vi "stupid get action.vi"(7 "transmit queue":refnum<queue>, 11 "application request in":T1) -> (0 "connection error":errorcluster)   [LabVIEW 2013]
uses:
  HTTP server/http request.ctl
  HTTP server/http method.ctl
  HTTP headers/http header data.ctl
  HTTP server/http response.ctl
  HTTP server/http response packet type.ctl
  HTTP server/Basic HTTP server.lvclass
  HTTP headers/http headers.lvlib
  HTTP responder/http responder.lvclass
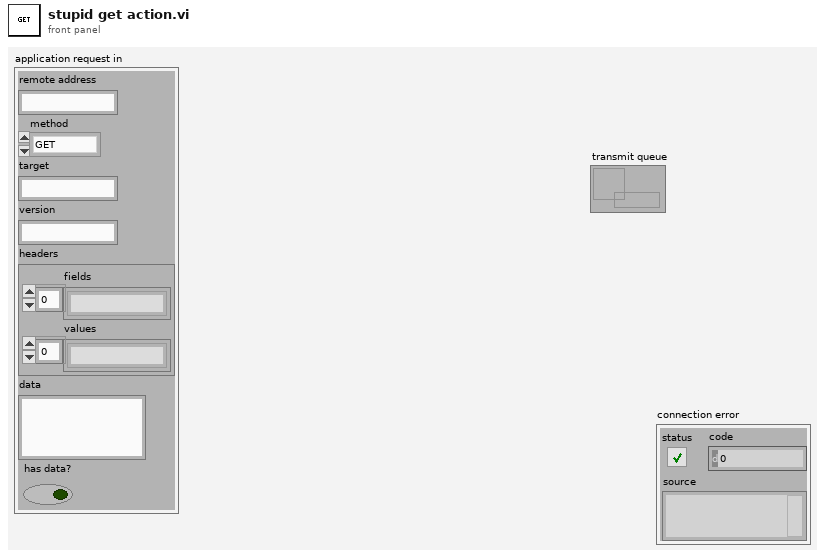
[diagram p1: front panel]
types:
  T1 = typedef "Basic HTTP server.lvclass/http request.ctl" = cluster{"remote address":string, "method":T2, "target":string, "version":string, "headers":T3, "data":string, "has data?":bool}
  T2 = typedef "Basic HTTP server.lvclass/http method.ctl" = enum16{"GET", "POST", "PUT", "DELETE", "HEAD", "OPTIONS", "upgrade"}
  T3 = typedef "http headers.lvlib/http header data.ctl" = cluster{"fields":string[], "values":string[]}
  T4 = typedef "Basic HTTP server.lvclass/http response packet type.ctl" = enum16{"full response", "header only", "data only", "last data"}
  T5 = typedef "Basic HTTP server.lvclass/http response.ctl" = cluster{"packet type":T4, "reason code":u16, "status string":string, "headers":T3, "cookies":string[], "data":string}
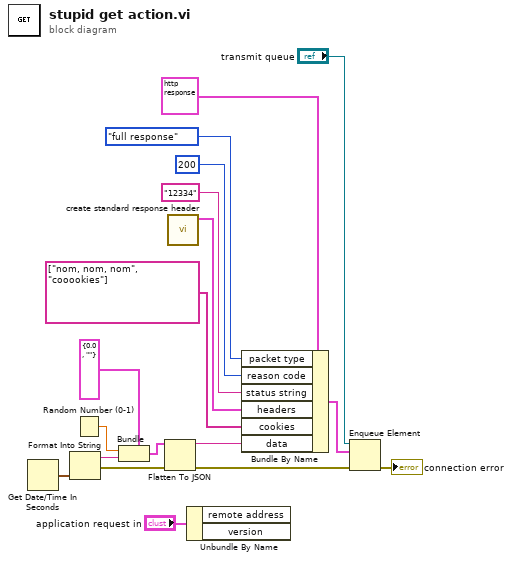
[diagram p0: block diagram]
diagram:
  n1 = Get Date/Time In Seconds() -> (seconds since 1Jan1904=w8:timestamp)
  n2 = Format Into String(w8) -> (resulting string=w5:string, error out=w9:errorcluster)  [unwired: 3 in]
  n3 = Random Number (0-1)() -> (number: 0 to 1=w3:dbl)
  n4 = Bundle(cluster=cluster{"n":dbl, "t":string} {"n"=0.0, "t"=""}, "n"=w3, "t"=w5) -> (w4:cluster{"n":dbl, "t":string})
  n5 = Flatten To JSON(anything=w4, error in (no error)=w9) -> (JSON string=w6:string, 11:w7:errorcluster)  [unwired: 1 in]
  n6 = call "create standard response header.vi"() -> ("default header"=w1:T3)  [unwired: 11 in]
  n7 = Unbundle By Name("application request in") -> ()  [unwired: 2 out]
  n8 = Bundle By Name(cluster=T5 {"packet type"=enum."full response", "reason code"=0, "status string"="", "headers"={"fields"=[], "values"=[]}, "cookies"=[], "data"=""} ("application request"), "packet type"=http_response_packet_type."full response", "reason code"=u16 200, "status string"="12334", "headers"=w1, "cookies"=string[] ["nom, nom, nom", "cooookies"], "data"=w6) -> (w11:T5)
  n9 = Enqueue Element(queue="transmit queue", element=w11, error in (no error)=w7) -> (error out=→"connection error":errorcluster)  [unwired: 1 in, 2 out]
